vi "conversion image monochrome.vi"(8 "error in (no error)":errorcluster caption="entrée d'erreur (pas d'erreur)", 11 "chemin du fichier (utiliser une boîte de dialogue)":path=path "C:/Documents and Settings/PROD/Bureau/Marion/Etiquettes emballage/logo FAS/logo FASmedic n&b.bmp") -> (0 "error out":errorcluster caption="sortie d'erreur", 1 "chaîne":string="ÿÿÿÿÿÿÿÿÿÿÿÿÿÿÿÿÿÿÿÿÿÿÿÿÿÿÿÿÿÿÿÿÿÿÿÿÿÿÿÿÿÿÿÿÿÿÿÿÿÿÿÿÿÿÿÿÿÿÿÿÿÿÿÿÿÿÿÿÿÿÿÿÿÿÿÿÿÿÿÿÿÿÿÿÿÿÿÿÿÿÿÿÿÿÿÿÿÿÿÿÿÿÿÿÿÿÿÿÿÿÿÿÿÿÿÿÿÿÿÿÿÿÿÿÿÿÿÿÿÿÿÿÿÿÿÿÿÿÿÿÿÿÿÿÿÿÿÿÿÿÿÿÿÿÿÿÿÿÿÿÿÿÿÿÿÿÿÿÿÿÿÿÿÿÿÿÿÿÿÿÿÿÿÿÿÿÿÿÿÿÿÿÿÿÿÿÿÿÿÿÿÿÿÿÿÿÿÿÿÿÿÿÿÿÿÿÿÿÿÿÿÿùÿÿÿÿÿÿÿÿÿÿÿÿÿÿÿÿÿÿÿÿÿÿÿÿÿÿÿÿÿÿÿÿÿÿÿÿÿÿÿÿÿÿÿÿÿÿÿÿÿÿÿÿÁÿÿÿÿÿÿÿÿÿÿÿÿÿÿÿÿÿÿÿÿÿÿÿÿÿÿÿÿÿÿÿÿÿÿÿÿÿÿÿÿÿÿÿÿÿÿÿÿÿÿÿÿ\u0000ÿÿÿÿÿÿÿÿÿÿÿÿÿÿÿÿÿÿÿÿÿÿÿÿÿÿÿÿÿÿÿÿÿÿÿÿÿÿÿÿÿÿÿÿÿÿÿÿÿÿÿø\u0000ÿÿÿÿÿÿÿÿÿÿÿÿÿÿÿÿÿÿÿÿÿÿÿÿÿÿÿÿÿÿÿÿÿÿÿÿÿÿÿÿÿÿÿÿÿÿÿÿÿÿÿà\u0000ÿÿÿÿÿÿÿÿÿÿÿÿÿÿÿÿÿÿÿÿÿÿÿÿÿÿÿÿÿÿÿÿÿÿÿÿÿÿÿÿÿÿÿÿÿÿÿÿÿÿ\u0000\u0000?ÿÿÿÿÿÿÿÿÿÿÿÿÿÿÿÿÿÿÿÿÿÿÿÿÿÿÿÿÿÿÿÿÿÿÿÿÿÿÿÿÿÿÿÿÿÿÿÿÿþ\u0000\u0000?ÿÿÿÿÿÿÿÿÿÿÿÿÿÿÿÿÿÿÿÿÿÿÿÿÿÿÿÿÿÿÿÿÿÿÿÿÿÿÿÿÿÿÿÿÿÿÿÿÿø\u0000\u0000?ÿÿÿÿÿ...", 2 "longueur V":i32=114, 3 "longueur H":i32=53)   [LabVIEW 2011]
uses:
  <vilib>/picture/picture.llb/imagedata.ctl
panel:
  out "1-bit pixmap":bool[][](array[boolean]) caption="table de pixels 1 bit"
  out "image data":T1={"image type"=0, "image depth"=1, "image"=array[6156 elements], "mask"=[], "colors"=[4278190080, 4294967295], "Rectangle"={"left"=0, "top"=0, "right"=424, "bottom"=114}} caption="données image"
  out "taille(s) 2":i32[](array[numeric])=[114, 424]
  out "Tableau 4":bool[](array[boolean])
  out "Tableau 3":bool[][](array[boolean])
  out "longueur chaine":i32=6042
  out "Tableau 2":bool[][](array[boolean])
  out "taille(s)":i32[](array[numeric])=[6042, 8]
  # "lignes"
  # "Colonnes"
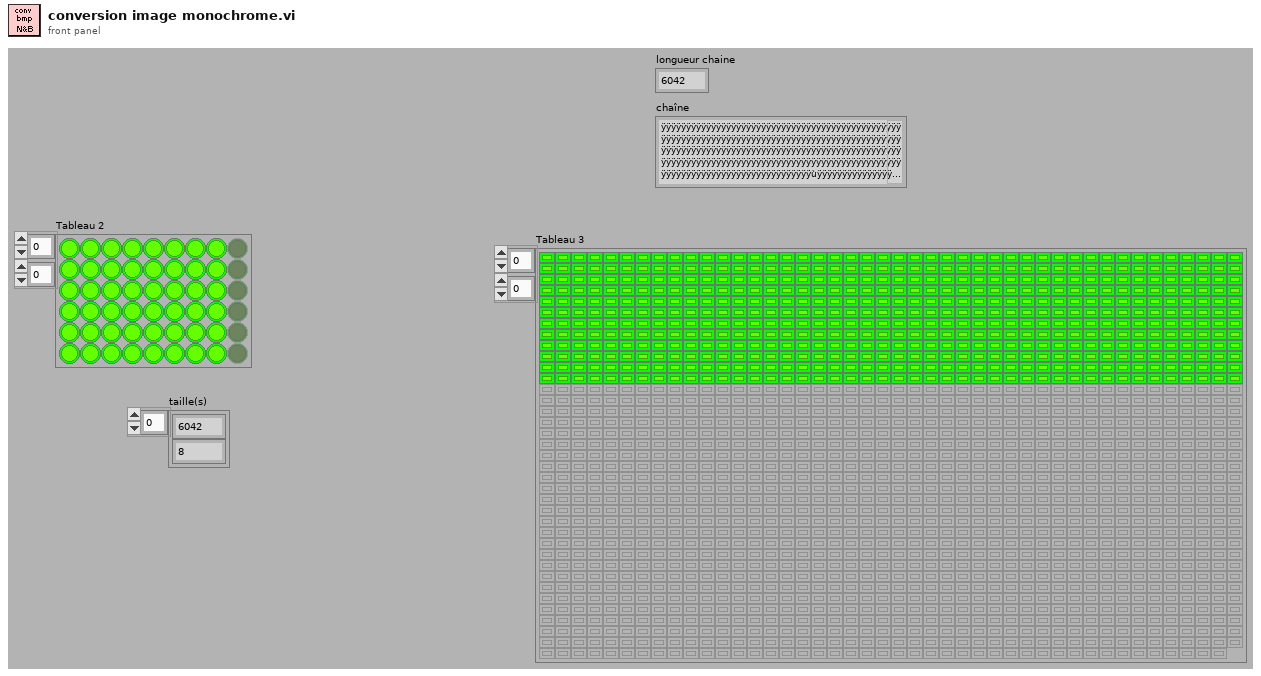
[diagram p1: front panel]
types:
  T1 = typedef "imagedata.ctl" = cluster{"image type":i32, "image depth":i32, "image":u8[], "mask":u8[], "colors":u32[], "Rectangle":cluster{"left":i16, "top":i16, "right":i16, "bottom":i16}}
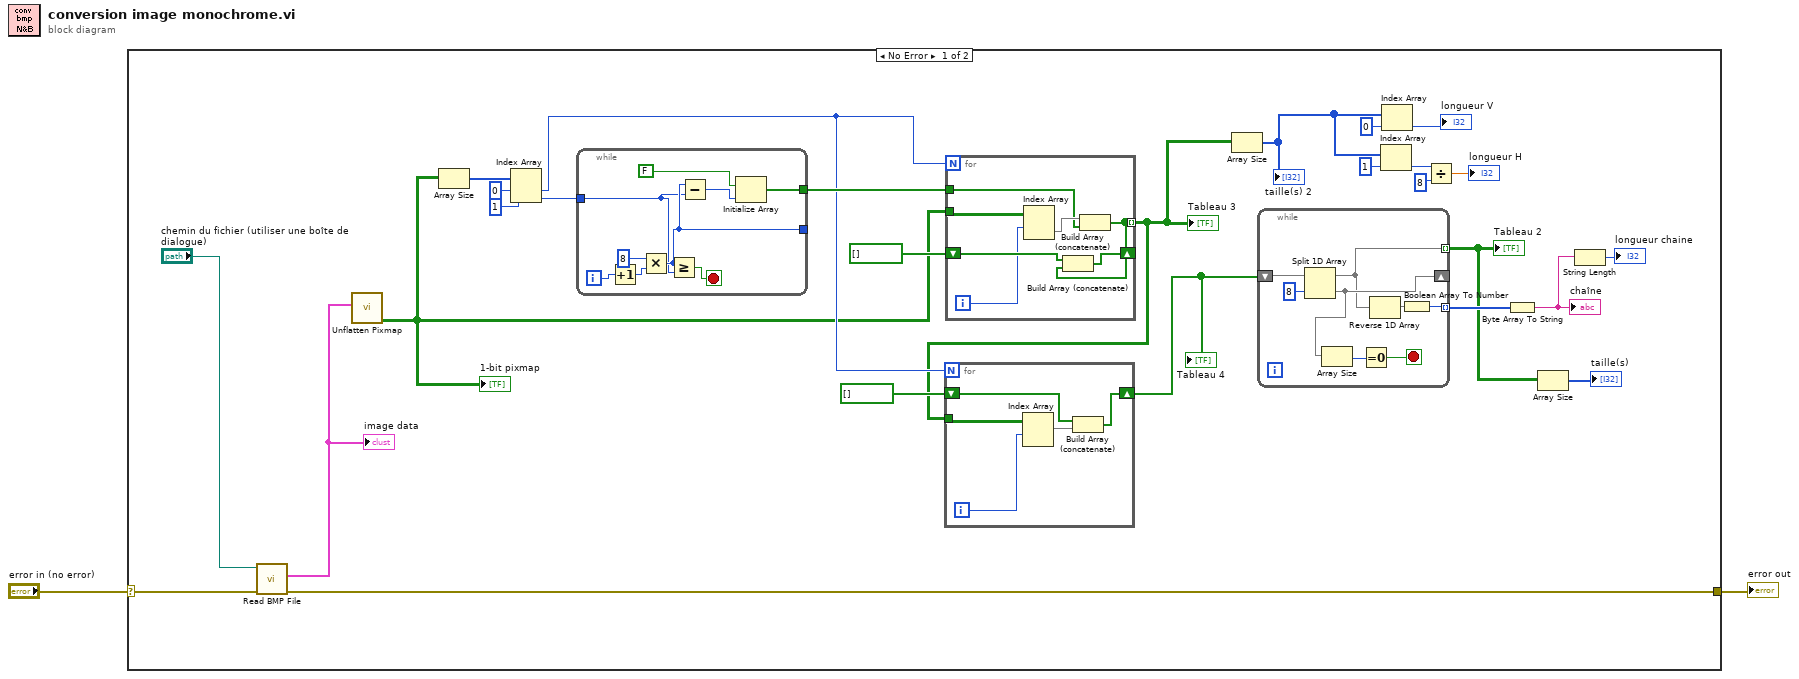
[diagram p0: block diagram]
diagram:
  n1 = case shown="No Error" "error in (no error)" {
    selector: "error in (no error)" -> [w4 w59]
    tunnel: [w3 w59] -> w1
    frame No Error {
      n2 = call <vilib>:"Read BMP File.vi"("error in (no error)"=w4, "path to BMP file"="chemin du fichier (utiliser une boîte de dialogue)") -> ("error out"=w3:errorcluster, "image data"=w14:T1)  [unwired: 7 in, 1 out]
      "image data" <- w14
      n3 = call <vilib>:"Unflatten Pixmap.vi"("image data"=w14) -> ("1-bit pixmap"=w13:bool[][])  [unwired: 4 in, 6 out]
      "1-bit pixmap" <- w13
      n4 = Array Size(array=w13) -> (size(s)=w24:i32[])
      n5 = Index Array(array=w24, index #1=0 ("indice"), index #2=1 ("indice")) -> (element #1=w18:i32, element #2=w19:i32)
      n6 = while {
        tunnel: w19 -> [w45]
        tunnel: [w46] -> _
        tunnel: [w42] -> w21
        i -> [w50]
        stop <- w47 stop-if-true
        n7 = Increment(x=w50) -> (x+1=w49:i32)
        n8 = Multiply(x=8, y=w49) -> (x*y=w46:i32)
        n9 = Greater Or Equal?(x=w46, y=w45) -> (x >= y?=w47:bool)
        n10 = Subtract(x=w46, y=w45) -> (x-y=w44:i32)
        n11 = Initialize Array(FALSE, w44) -> (w42:bool[])
      }
      n12 = for {
        N: w18 -> [_]
        tunnel: w13 -> [w41]
        tunnel: w21 -> [w39]
        tunnel: [w38] -> w16 mode=indexing
        shift-right: [w37] -> _
        shift-left: bool[] [] -> [w36]
        i -> [w35]
        n13 = Index Array(array=w41, index (row)=w35) -> (element=w40:bool[])  [unwired: 1 in]
        n14 = Build Array (concatenate)(w40, w39) -> (w38:bool[])
        n15 = Build Array (concatenate)(w36, w38) -> (w37:bool[])
      }
      "Tableau 3" <- w16
      n16 = for {
        N: w18 -> [_]
        tunnel: w16 -> [w34]
        shift-right: [w33] -> w12
        shift-left: bool[] [] -> [w32]
        i -> [w31]
        n17 = Index Array(array=w34, index (row)=w31) -> (element=w30:bool[])  [unwired: 1 in]
        n18 = Build Array (concatenate)(w32, w30) -> (w33:bool[])
      }
      "Tableau 4" <- w12
      n19 = Array Size(array=w16) -> (size(s)=w11:i32[])
      "taille(s) 2" <- w11
      n20 = while {
        tunnel: [w51] -> w28 mode=indexing
        shift-right: [w52] -> _
        shift-left: w12 -> [w58]
        tunnel: [w54] -> w29 mode=indexing
        stop <- w56 stop-if-true
        n21 = Split 1D Array(array=w58, index=8 ("indice")) -> (first subarray=w51:bool[], second subarray=w52:bool[])
        n22 = Array Size(array=w52) -> (size(s)=w55:i32)
        n23 = Equal To 0?(x=w55) -> (x = 0?=w56:bool)
        n24 = Reverse 1D Array(array=w51) -> (reversed array=w53:bool[])
        n25 = Boolean Array To Number(Boolean array=w53) -> (number=w54:u32)
      }
      "Tableau 2" <- w28
      n26 = Index Array(array=w11, index=1 ("indice")) -> (element=w8:i32)
      n27 = Index Array(array=w11, index=0 ("indice")) -> (element=→"longueur V":i32)
      n28 = Divide(x=w8, y=8) -> (x/y=→"longueur H":dbl)
      n29 = Byte Array To String(unsigned byte array=w29) -> (string=w26:string)
      "chaîne" <- w26
      n30 = Array Size(array=w28) -> (size(s)=→"taille(s)":i32[])
      n31 = String Length(string=w26) -> (length=→"longueur chaine":i32)
    }
    frame Error {
    }
  }
  "error out" <- w1
